vi "prueba 2.vi"() -> ()   [LabVIEW 2014]
uses:
  <vilib>/addons/database/Auxilliary.llb/DB Tools Column Info.ctl
  <vilib>/addons/database/Auxilliary.llb/DB Tools DataTypes.ctl
  SEQ/SeqLoop/TypeDefs/HW InOut MAP.ctl
  <vilib>/addons/database/NI_Database_API.lvlib
  SEQ/SeqLoop/SeqLoop.lvlib
panel:
  out "tables 2":string[](array[string])
  out "error out":errorcluster
  in  "Enum":T1(ring)
  in  "table":string="win1"
  in  "error in (no error)":errorcluster
  out "data":string[][](array[string])
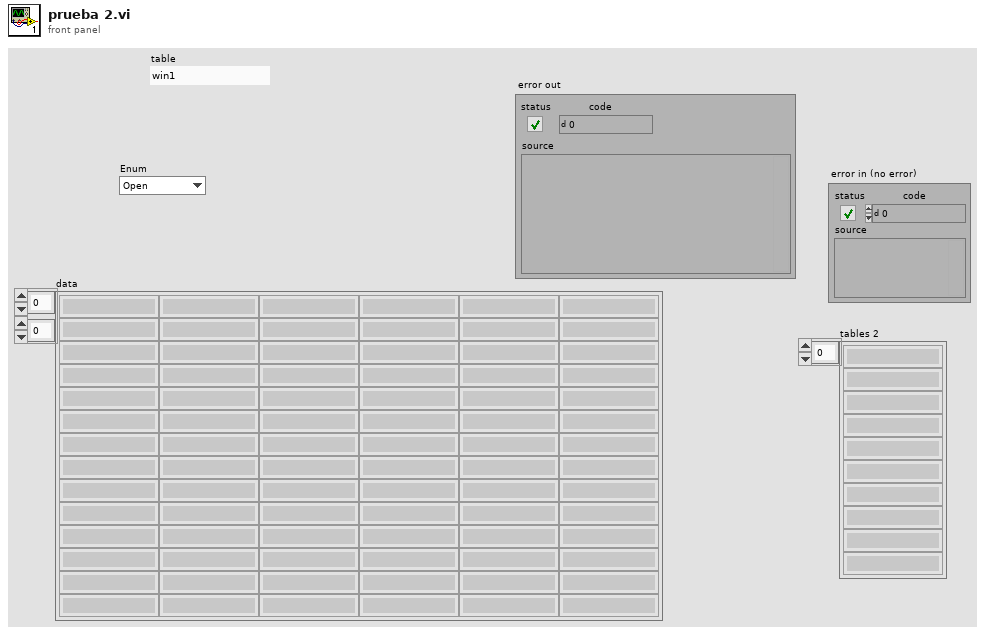
[diagram p1: front panel]
types:
  T1 = enum16{"Open", "Create", "Delete", "Read_HAL", "Read_CORE", "Read_UI", "Read_MATH", "Read_SEQ", "Write_HAL", "Write_CORE", "Write_UI", "Write_MATH", "Write_SEQ", "Close"}
  T2 = typedef "SeqLoop.lvlib/HW InOut MAP.ctl" = cluster{"Inputs":cluster{"Entrada":i32, "Descripción":string, "Habilitada?":bool}[][], "Outputs":cluster{"Salida":i32, "Descripción":string, "Habilitada?":bool, "Formula":string, "Tipo de Salida":string}[][]}
  T3 = typedef "NI_Database_API.lvlib/DB Tools Column Info.ctl" = cluster{"column name":string, "data type":T4, "size":i32, "allow null?":bool}
  T4 = typedef "NI_Database_API.lvlib/DB Tools DataTypes.ctl" = enum16{"String", "Long (I32)", "Single (SGL)", "Double (DBL)", "Date/Time", "Binary"}
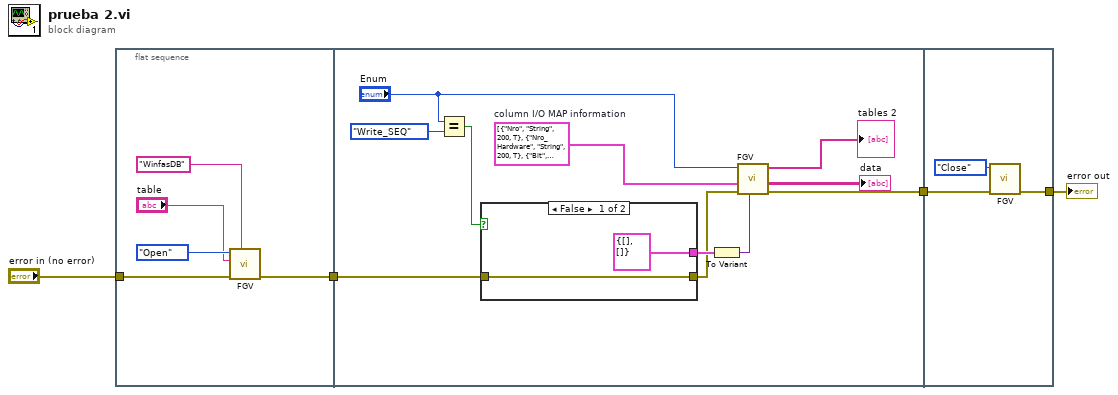
[diagram p0: block diagram]
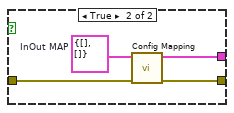
[diagram p2: hidden frame]
diagram:
  n1 = flat-sequence {
    tunnel: "error in (no error)" -> [w9]
    tunnel: [w8] -> w3
    tunnel: [w12] -> w1
    tunnel: w3 -> [w17]
    tunnel: [w29] -> w2
    tunnel: w1 -> [w28]
    frame #0 {
      n2 = call "FGV.vi"("Connection Information"="WinfasDB", "error in (no error)"=w9, "table"="table", "Enum"=T1."Open") -> ("error out"=w8:errorcluster)  [unwired: 5 in, 2 out]
    }
    frame #1 {
      w13 = T3[] [{"column name"="Nro", "data type"=enum."String", "size"=200, "allow null?"=TRUE}, {"column name"="Nro_Hardware", "data type"=enum."String", "size"=200, "allow null?"=TRUE}, {"column name"="Bit", "data type"=enum."String", "size"=200, "allow null?"=TRUE}, {"column name"="Descripcion", "data type"=enum."String", "size"=200, "allow null?"=TRUE}, {"column name"="Habilitada", "data type"=enum."String", "size"=200, "allow null?"=TRUE}]  # column I/O MAP information
      n3 = Equal?(x="Enum", y=T1."Write_SEQ") -> (x = y?=w14:bool)
      n4 = case shown="False" w14 {
        tunnel: [T2 {"Inputs"=[], "Outputs"=[]} ("HW InOut MAP out") w26] -> w20
        tunnel: [w22 w25] -> w18
        tunnel: w17 -> [w22 w24]
        frame False {
        }
        frame True {
          w23 = T2 {"Inputs"=[], "Outputs"=[]}  # InOut MAP
          n5 = call "Config Mapping.vi"("error in (no error)"=w24, "HW InOut MAP in"=w23) -> ("error out"=w25:errorcluster, "HW InOut MAP out"=w26:T2)  [unwired: 8 in]
        }
      }
      n6 = To Variant(anything=w20) -> (Variant=w19:variant)
      n7 = call "FGV.vi"("Variant"=w19, "error in (no error)"=w18, "column information"=w13, "Enum"="Enum") -> ("error out"=w12:errorcluster, "data"=→"data":string[][], "tables"=→"tables 2":string[])  [unwired: 5 in]
    }
    frame #2 {
      n8 = call "FGV.vi"("error in (no error)"=w28, "Enum"=T1."Close") -> ("error out"=w29:errorcluster)  [unwired: 7 in, 2 out]
    }
  }
  "error out" <- w2
